vi "Get position.vi"(8 "error in (no error)":errorcluster, 11 "MotorSim in":refnum<class "MotorSim.lvclass">) -> (0 "error out":errorcluster, 1 "end":bool, 2 "simulated position":i32, 3 "MotorSim out":refnum<class "MotorSim.lvclass">, 4 "current position":string)   [LabVIEW 2018, in "MotorSim.lvclass"]
uses:
  MotorSim.lvclass
  MotorSim.lvclass/MotorSim.ctl
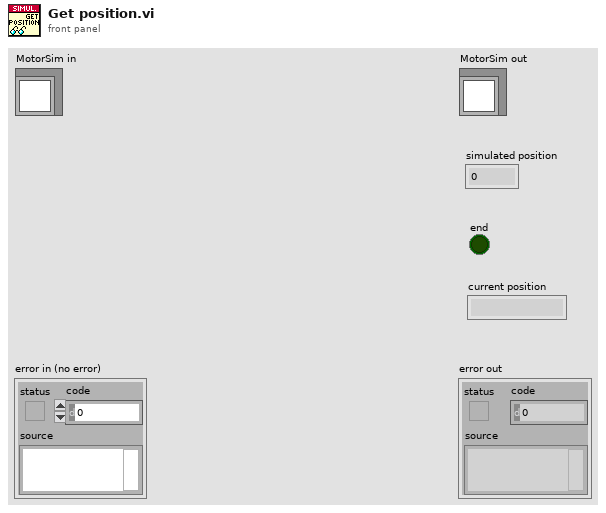
[diagram p1: front panel]
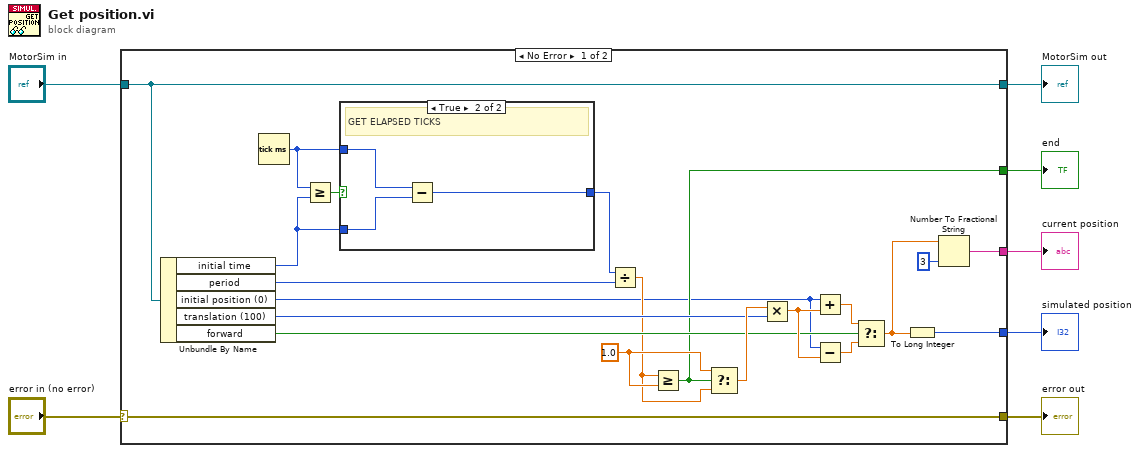
[diagram p0: block diagram]
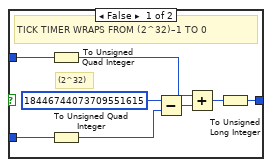
[diagram p2: hidden frame]
diagram:
  n1 = case shown="No Error" "error in (no error)" {
    selector: "error in (no error)" -> [w28 w40]
    tunnel: [w28 w40] -> w6
    tunnel: [w27 w41] -> w4
    tunnel: "MotorSim in" -> [w27 w41]
    tunnel: [w15 _] -> w3
    tunnel: [w14 _] -> w2
    tunnel: [w13 _] -> w1
    frame No Error {
      w21 = 1.0 ("x")
      n2 = Unbundle By Name(w27) -> ("initial time"=w19:u32, "period"=w18:u32, "initial position (0)"=w10:i32, "translation (100)"=w16:i32, "forward"=w17:bool)
      n3 = Tick Count (ms)() -> (millisecond timer value=w26:u32)
      n4 = Greater Or Equal?(x=w26, y=w19) -> (x >= y?=w11:bool)
      n5 = case shown="True" w11 {
        tunnel: w19 -> [w36 w38]
        tunnel: w26 -> [w33 w39]
        tunnel: [w32 w37] -> w25
        frame False {
          # "(2^32)"
          # "TICK TIMER WRAPS FROM (2^32)–1 TO 0"
          n6 = To Unsigned Quad Integer(1:w33) -> (0:w30:u64)
          n7 = To Unsigned Quad Integer(1:w36) -> (0:w35:u64)
          n8 = Subtract(x=u64 18446744073709551615 ("initial Tick"), y=w35) -> (x-y=w29:u64)
          n9 = Add(x=w30, y=w29) -> (x+y=w31:u64)
          n10 = To Unsigned Long Integer(number=w31) -> (unsigned 32bit integer=w32:u32)
        }
        frame True {
          # "GET ELAPSED TICKS"
          n11 = Subtract(x=w39, y=w38) -> (x-y=w37:u32)
        }
      }
      n12 = Divide(x=w25, y=w18) -> (x/y=w12:dbl)
      n13 = Greater Or Equal?(x=w12, y=w21) -> (x >= y?=w15:bool)
      n14 = Select(t=w21, s=w15, f=w12) -> (s? t:f=w20:dbl)
      n15 = Multiply(x=w20, y=w16) -> (x*y=w24:dbl)
      n16 = Add(x=w10, y=w24) -> (x+y=w22:dbl)
      n17 = Subtract(x=w10, y=w24) -> (x-y=w23:dbl)
      n18 = Select(t=w22, s=w17, f=w23) -> (s? t:f=w9:dbl)
      n19 = To Long Integer(number=w9) -> (32bit integer=w13:i32)
      n20 = Number To Fractional String(number=w9, precision (6)=i16 3) -> (F-format string=w14:string)  [unwired: 2 in]
    }
    frame Error {
    }
  }
  "error out" <- w6
  "MotorSim out" <- w4
  "end" <- w3
  "current position" <- w2
  "simulated position" <- w1
